vi "SubVI_EXA frequency.vi"(6 "SPAN Unit":u16(ring) items=["Hz", "kHz", "MHz", "GHz"], 7 "CENTRE F Unit":u16(ring) items=["Hz", "kHz", "MHz", "GHz"], 8 "error in (no error)":errorcluster, 9 "Span":dbl, 10 "Centre Frequency":dbl, 11 "VISA Refnum in":refnum<visa-resource-name>) -> (0 "error out":errorcluster, 3 "VISA resource name":refnum<visa-resource-name>)   [LabVIEW 2016]
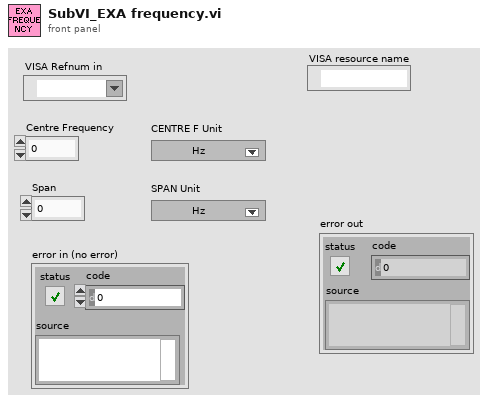
[diagram p1: front panel]
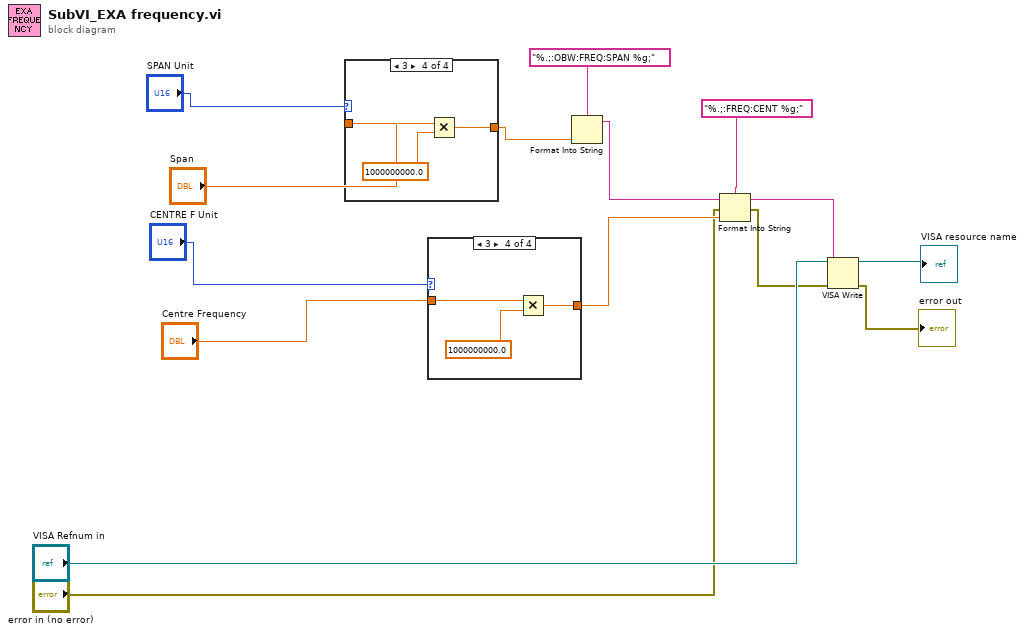
[diagram p0: block diagram]
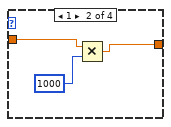
[diagram p3: hidden frame]
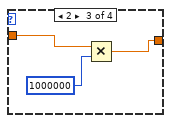
[diagram p4: hidden frame]
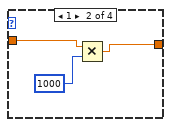
[diagram p6: hidden frame]
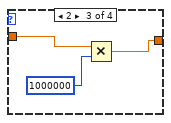
[diagram p7: hidden frame]
diagram:
  n1 = case shown="3" "SPAN Unit" {
    tunnel: [w16 w17 w20 w23] -> w12
    tunnel: "Span" -> [w16 w19 w22 w24]
    frame 0, Default {
    }
    frame 1 {
      n2 = Multiply(x=w19, y=1000) -> (x*y=w17:dbl)
    }
    frame 2 {
      n3 = Multiply(x=w22, y=1000000) -> (x*y=w20:dbl)
    }
    frame 3 {
      n4 = Multiply(x=w24, y=1000000000.0) -> (x*y=w23:dbl)
    }
  }
  n5 = case shown="3" "CENTRE F Unit" {
    tunnel: [w26 w27 w30 w34] -> w14
    tunnel: "Centre Frequency" -> [w26 w29 w32 w33]
    frame 0, Default {
    }
    frame 1 {
      n6 = Multiply(x=w29, y=1000) -> (x*y=w27:dbl)
    }
    frame 2 {
      n7 = Multiply(x=w32, y=1000000) -> (x*y=w30:dbl)
    }
    frame 3 {
      n8 = Multiply(x=w33, y=1000000000.0) -> (x*y=w34:dbl)
    }
  }
  n9 = Format Into String(format string="%.;:OBW:FREQ:SPAN %g;", w12) -> (resulting string=w11:string)  [unwired: 2 in, 1 out]
  n10 = Format Into String(format string="%.;:FREQ:CENT %g;", initial string=w11, error in="error in (no error)", w14) -> (resulting string=w5:string, error out=w6:errorcluster)
  n11 = VISA Write(VISA resource name="VISA Refnum in", write buffer=w5, error in (no error)=w6) -> (VISA resource name out=→"VISA resource name":refnum<visa-resource-name>, error out=→"error out":errorcluster)  [unwired: 1 out]
